vi "TRITON_TEMP_LOCKED.vi"(1 "Temperature Control Spec":dbl, 2 "Target Temperature":dbl, 3 "Temperature Data Array":dbl[](array[numeric])) -> (0 "Locked on Setpoint?":bool)   [LabVIEW 2009]
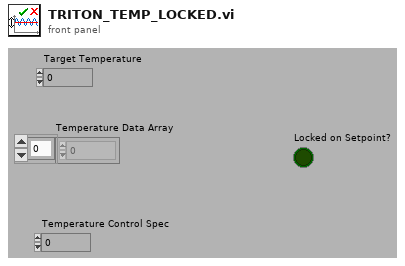
[diagram p1: front panel]
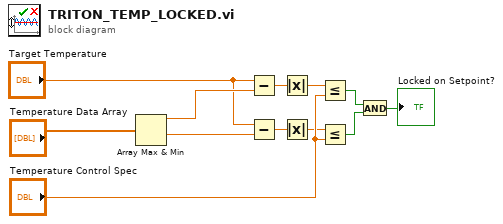
[diagram p0: block diagram]
diagram:
  n1 = Array Max & Min(array="Temperature Data Array") -> (max value=w11:dbl, min value=w9:dbl)  [unwired: 2 out]
  n2 = Subtract(x="Target Temperature", y=w11) -> (x-y=w10:dbl)
  n3 = Subtract(x="Target Temperature", y=w9) -> (x-y=w8:dbl)
  n4 = Absolute Value(x=w10) -> (abs(x)=w6:dbl)
  n5 = Absolute Value(x=w8) -> (abs(x)=w4:dbl)
  n6 = Less Or Equal?(x=w6, y="Temperature Control Spec") -> (x <= y?=w2:bool)
  n7 = Less Or Equal?(x=w4, y="Temperature Control Spec") -> (x <= y?=w3:bool)
  n8 = And(x=w2, y=w3) -> (x .and. y?=→"Locked on Setpoint?":bool)
